vi "Sync.vi"(6 "timeout(10s)":u32=10, 8 "error in (no error)":errorcluster) -> (0 "error out":errorcluster, 1 "timeout?":bool)   [LabVIEW 2017, in "MDPtr.lvlib" / "MDPtrMgr.lvclass"]
uses:
  MDPtrMgr.lvclass
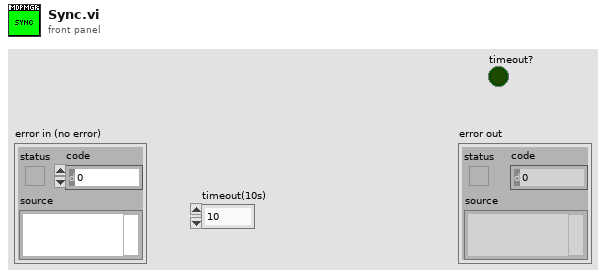
[diagram p1: front panel]
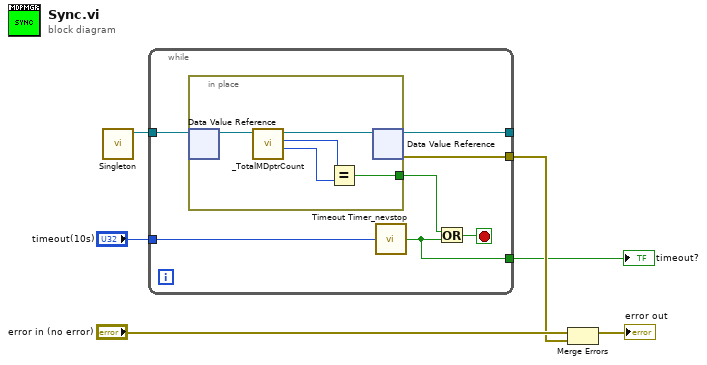
[diagram p0: block diagram]
diagram:
  n1 = call "Singleton.vi"() -> ("MDPtrMgrDVR"=w1:refnum<data-value>)  [unwired: 10 in, 1 out]
  n2 = while {
    tunnel: w1 -> [w13]
    tunnel: [w12] -> w4
    tunnel: "timeout(10s)" -> [w11]
    tunnel: [w8] -> w2
    tunnel: [w7] -> _
    stop <- w9 stop-if-true
    n3 = in-place {
      in-place-border: [w14] -> w10
      n4 = in-place-dvr #1(w13) -> (w18:refnum<class "MDPtrMgr.lvclass">)  [unwired: 1 out]
      n5 = call "_TotalMDptrCount.vi"("MDPtrMgr in"=w18) -> ("# free elements in queue"=w15:i32, "# elements in queue"=w16:i32, "MDPtrMgr out"=w17:refnum<class "MDPtrMgr.lvclass">)  [unwired: 6 in, 2 out]
      n6 = Equal?(x=w16, y=w15) -> (x = y?=w14:bool)
      n7 = in-place-dvr #1(w17) -> (w7:refnum<data-value>, w12:errorcluster)
    }
    n8 = call <userlib>:"Timeout Timer_nevstop.vi"("timeout(s)"=w11) -> ("timeout?"=w8:bool)  [unwired: 7 in, 1 out]
    n9 = Or(x=w10, y=w8) -> (x .or. y?=w9:bool)
  }
  "timeout?" <- w2
  n10 = Merge Errors("error in (no error)", w4) -> (→"error out":errorcluster)
